vi "Calibration Delete Parameters.vi"(8 "error in (no error)":errorcluster, 10 "VariableName":string, 11 "Main":string="0") -> (0 "error out":errorcluster)   [LabVIEW 2017, in "SQLite.lvclass"]
doc: "delete the parameters in calibration DB.\nVariableName accept multi lines string.\n\n2016-03-17 10:23:18\n蒋松\nsina: @sushu1051"
uses:
  SQLite.lvclass
  SQLiteFileName.ctl
  TabelFullName.ctl
  <userlib>/LabSQL/LabSQL.lvlib
  <userlib>/sushu/sushu.lvlib
panel:
  out "Select SQL CMD":string
  # "132423"
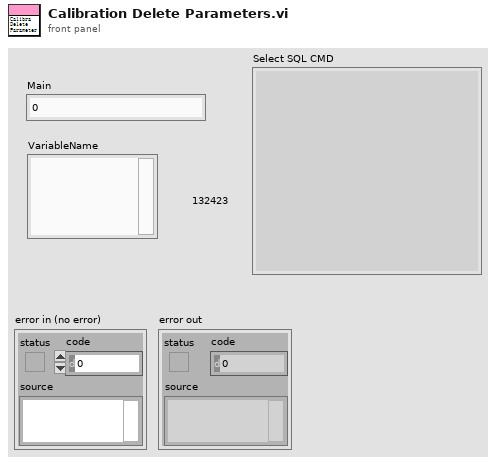
[diagram p1: front panel]
types:
  T1 = typedef "SQLite.lvclass/TabelFullName.ctl" = string
  T2 = typedef "SQLite.lvclass/SQLiteFileName.ctl" = string
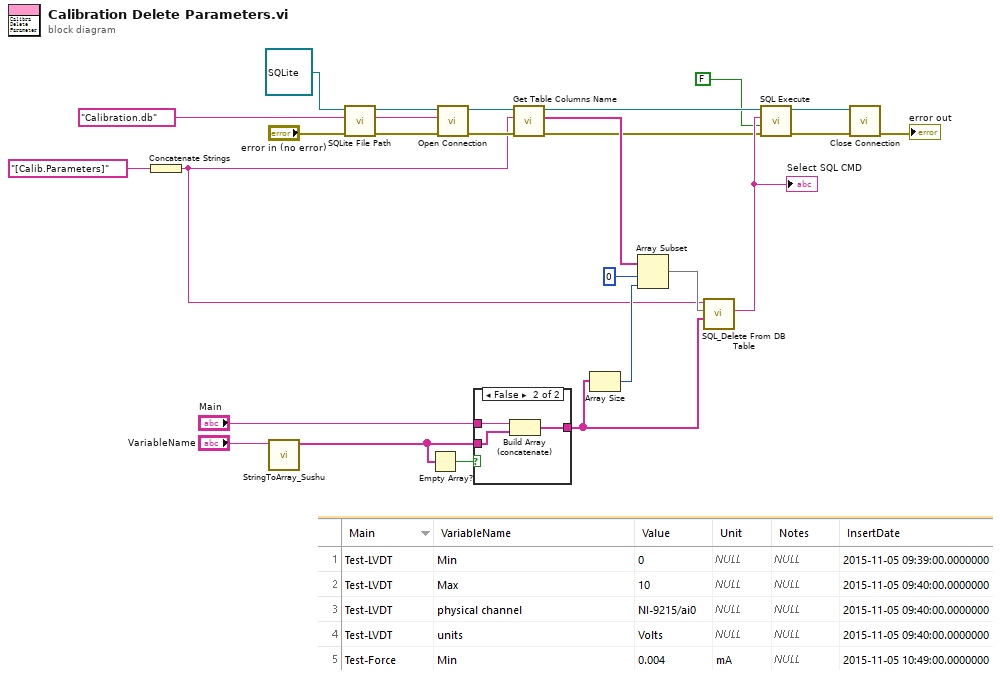
[diagram p0: block diagram]
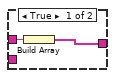
[diagram p2: hidden frame]
diagram:
  n1 = Concatenate Strings(T1 "[Calib.Parameters]" ("TabelFullName")) -> (w2:string)
  n2 = call <userlib>:"StringToArray_Sushu.vi"("State Queue"="VariableName") -> ("Array"=w24:string[])  [unwired: 8 in, 2 out]
  n3 = call "SQLite File Path.vi"("error in (no error)"="error in (no error)", "SQLiteFileName"=T2 "Calibration.db", "SQLite in"=refnum<class "SQLite.lvclass"> refnum ("SQLite.lvclass")) -> ("error out"=w3:errorcluster, "string"=w21:string, "SQLite out"=w19:refnum<class "SQLite.lvclass">)  [unwired: 6 in]
  n4 = Empty Array?(array=w24) -> (empty?=w14:bool)
  n5 = call-dynamic "Open Connection.vi"("error in (no error)"=w3, "ConnectionString"=w21, "HostDB in"=w19) -> ("error out"=w22:errorcluster, "HostDB out"=w23:refnum<class "SQLite.lvclass">)  [unwired: 7 in]
  n6 = case shown="False" w14 {
    tunnel: "Main" -> [w28 w31]
    tunnel: [w27 w30] -> w18
    tunnel: w24 -> [_ w29]
    frame True {
      n7 = Build Array(w28) -> (w27:string[])
    }
    frame False {
      n8 = Build Array (concatenate)(w31, w29) -> (w30:string[])
    }
  }
  n9 = call-dynamic "Get Table Columns Name.vi"("error in (no error)"=w22, "TableName"=w2, "HostDB in"=w23) -> ("error out"=w5:errorcluster, "ColunmsList"=w11:string[], "HostDB out"=w10:refnum<class "SQLite.lvclass">)  [unwired: 4 in, 2 out]
  n10 = Array Size(array=w18) -> (size(s)=w16:i32)
  n11 = Array Subset(array=w11, index=0, length=w16) -> (w15:string[])
  n12 = call <userlib>:"SQL_Delete From DB Table.vi"("ColumnsValue"=w18, "ColumnsNameList"=w15, "TableName"=w2) -> ("Select SQL CMD"=w9:string)  [unwired: 8 in]
  "Select SQL CMD" <- w9
  n13 = call-dynamic "SQL Execute.vi"("error in (no error)"=w5, "Return Data (T)"=FALSE, "Command Text"=w9, "HostDB in"=w10) -> ("error out"=w6:errorcluster, "HostDB out"=w7:refnum<class "SQLite.lvclass">)  [unwired: 3 in, 3 out]
  n14 = call-dynamic "Close Connection.vi"("error in (no error)"=w6, "HostDB in"=w7) -> ("error out"=→"error out":errorcluster)  [unwired: 8 in, 1 out]
